vi "pulseFinishing.vi"(8 "error in (no error)":errorcluster, 11 "ScriptEventList in":refnum<class "ScriptEventList.lvclass">) -> (0 "error out":errorcluster, 3 "ScriptEventList out":refnum<class "ScriptEventList.lvclass">)   [LabVIEW 2009, in "Tools.lvlib" / "Scripting.lvlib" / "ScriptEventList.lvclass"]
uses:
  ScriptEventList.lvclass
  ScriptEvent.lvclass
  ScriptEventList.lvclass/ScriptEventList.ctl
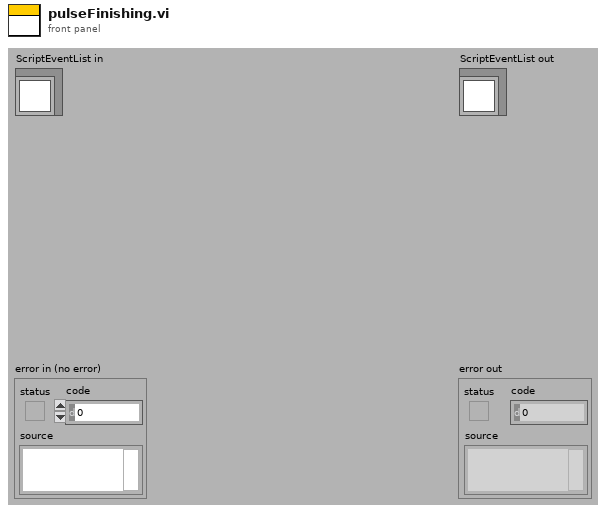
[diagram p1: front panel]
types:
  T1 = enum16{"changeValue", "pulse", "clock", "rampUp", "rampDown", "singleTone", "singleToneRamp", "playFile", "rf", "rfRamp"}
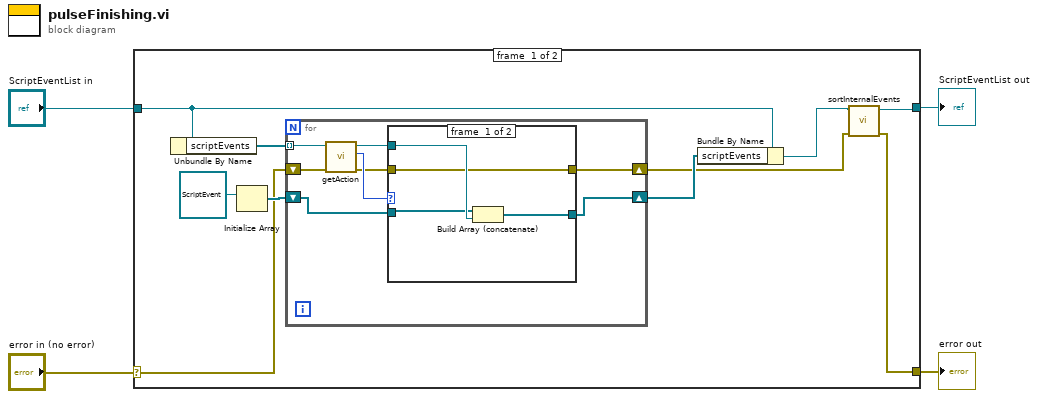
[diagram p0: block diagram]
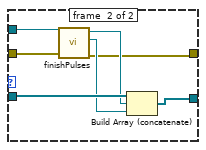
[diagram p2: hidden frame]
diagram:
  n1 = case shown="No Error" "error in (no error)" {
    selector: "error in (no error)" -> [w11 w35]
    tunnel: [w5 w35] -> w3
    tunnel: [w10 w34] -> w1
    tunnel: "ScriptEventList in" -> [w8 w34]
    frame #0 {
      n2 = Unbundle By Name(w8) -> ("scriptEvents"=w14:refnum<class "ScriptEvent.lvclass">[])
      n3 = Initialize Array(refnum<class "ScriptEvent.lvclass"> refnum ("Tools.lvlib:Scripting.lvlib:ScriptEvent.lvclass")) -> (w12:refnum<class "ScriptEvent.lvclass">[])  [unwired: 1 in]
      n4 = for {
        tunnel: w14 -> [w22] mode=indexing
        shift-right: [w16] -> w9
        shift-left: w12 -> [w17]
        shift-right: [w15] -> w6
        shift-left: w11 -> [w21]
        n5 = call "getAction.vi"("error in (no error)"=w21, "ScriptEvent.lvclass in"=w22) -> ("error out"=w19:errorcluster, "action"=w20:T1, "ScriptEvent.lvclass out"=w18:refnum<class "ScriptEvent.lvclass">)  [unwired: 7 in]
        n6 = case shown="\"pulse\"" w20 {
          tunnel: w19 -> [w23 w32]
          tunnel: w18 -> [w26 w33]
          tunnel: w17 -> [w25 w31]
          tunnel: [w24 w27] -> w16
          tunnel: [w23 w28] -> w15
          frame #0 {
            n7 = Build Array (concatenate)(w25, w26) -> (w24:refnum<class "ScriptEvent.lvclass">[])
          }
          frame #1 {
            n8 = call "finishPulses.vi"("error in (no error)"=w32, "ScriptEvent in"=w33) -> ("error out"=w28:errorcluster, "pulse finish"=w29:refnum<class "ScriptEvent.lvclass">, "ScriptEvent out"=w30:refnum<class "ScriptEvent.lvclass">)  [unwired: 7 in]
            n9 = Build Array (concatenate)(w31, w30, w29) -> (w27:refnum<class "ScriptEvent.lvclass">[])
          }
        }
      }
      n10 = Bundle By Name(cluster=w8, "scriptEvents"=w9) -> (w7:refnum<class "ScriptEventList.lvclass">)
      n11 = call "sortInternalEvents.vi"("error in (no error)"=w6, "ScriptEventList in"=w7) -> ("error out"=w5:errorcluster, "ScriptEventList out"=w10:refnum<class "ScriptEventList.lvclass">)  [unwired: 8 in]
    }
    frame #1 {
    }
  }
  "error out" <- w3
  "ScriptEventList out" <- w1
